vi "meth.PushCluster.vi"(0 "class.GLue in":refnum<class "class.GLue.lvclass">, 7 "Cluster":variant, 11 "error in":errorcluster) -> (4 "class.GLue out":refnum<class "class.GLue.lvclass">, 8 "Pushed?":bool=TRUE, 15 "error out":errorcluster)   [LabVIEW 2014, in "GLue.lvlib" / "class.GLue.lvclass"]
uses:
  class.GLue.lvclass
  class.GLue.lvclass/class.GLue.ctl
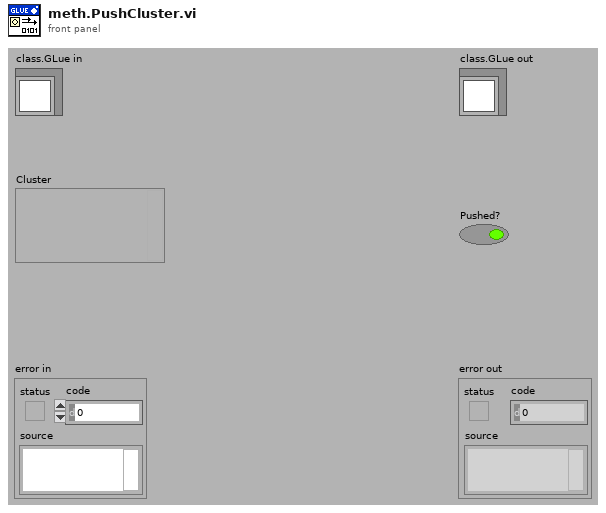
[diagram p1: front panel]
types:
  T1 = cluster{"length":u16, "private":u8, "type":enum8{"<Null>", "I8", "I16", "I32", "I64", "U8", "U16", "U32", "U64", "SGL", "DBL", "EXT", "CSG", "CDB", "CXT", "0x0F", "0x10", "0x11", "0x12", "0x13", "0x14", "Enum U8", "Enum U16", "Enum U32", "Enum U64", "SGL PQ", "DBL PQ", "EXT PQ", "CSG PQ", "CDB PQ", "CXT PQ", "0x1F", "0x20", "Boolean", "0x22", "0x23", "0x24", "0x25", "0x26", "0x27", "0x28", "0x29", "0x2A", "0x2B", "0x2C", "0x2D", "0x2E", "0x2F", "String", "0x31", "Path", "Pict", "0x34", "0x35", "0x36", "DAQ", "0x38", "0x39", "0x3A", "0x3B", "0x3C", "0x3D", "0x3E", "0x3F", "Array", "0x41", "0x42", "0x43", "0x44", "0x45", "0x46", "0x47", "0x48", "0x49", "0x4A", "0x4B", "0x4C", "0x4D", "0x4E", "0x4F", "Cluster", "0x51", "0x52", "Variant", "Waveform", "0x55", "0x56", "0x57", "0x58", "0x59", "0x5A", "0x5B", "0x5C", "0x5D", "0x5E", "0x5F", "0x60", "0x61", "0x62", "0x63", "0x64", "0x65", "0x66", "0x67", "0x68", "0x69", "0x6A", "0x6B", "0x6C", "0x6D", "0x6E", "0x6F", "Refnum"}, "# elements":u16}
  T2 = enum8{"<Null>", "I8", "I16", "I32", "I64", "U8", "U16", "U32", "U64", "SGL", "DBL", "EXT", "CSG", "CDB", "CXT", "0x0F", "0x10", "0x11", "0x12", "0x13", "0x14", "Enum U8", "Enum U16", "Enum U32", "Enum U64", "SGL PQ", "DBL PQ", "EXT PQ", "CSG PQ", "CDB PQ", "CXT PQ", "0x1F", "0x20", "Boolean", "0x22", "0x23", "0x24", "0x25", "0x26", "0x27", "0x28", "0x29", "0x2A", "0x2B", "0x2C", "0x2D", "0x2E", "0x2F", "String", "0x31", "Path", "Pict", "0x34", "0x35", "0x36", "DAQ", "0x38", "0x39", "0x3A", "0x3B", "0x3C", "0x3D", "0x3E", "0x3F", "Array", "0x41", "0x42", "0x43", "0x44", "0x45", "0x46", "0x47", "0x48", "0x49", "0x4A", "0x4B", "0x4C", "0x4D", "0x4E", "0x4F", "Cluster", "0x51", "0x52", "Variant", "Waveform", "0x55", "0x56", "0x57", "0x58", "0x59", "0x5A", "0x5B", "0x5C", "0x5D", "0x5E", "0x5F", "0x60", "0x61", "0x62", "0x63", "0x64", "0x65", "0x66", "0x67", "0x68", "0x69", "0x6A", "0x6B", "0x6C", "0x6D", "0x6E", "0x6F", "Refnum"}
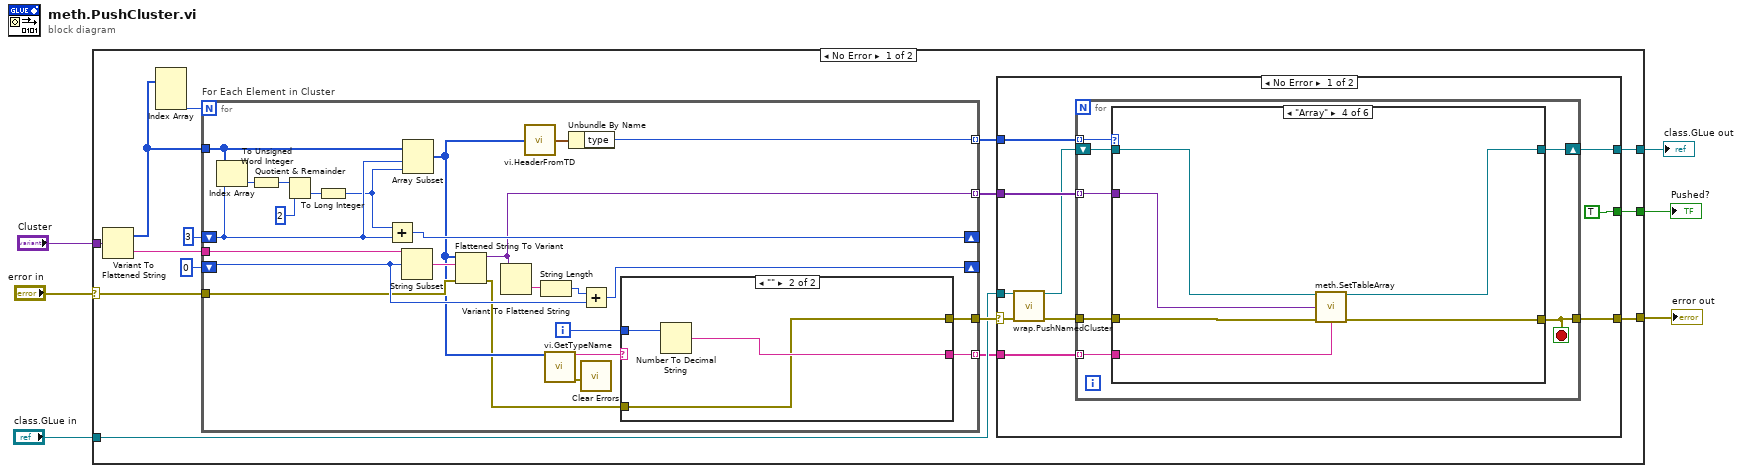
[diagram p0: block diagram]
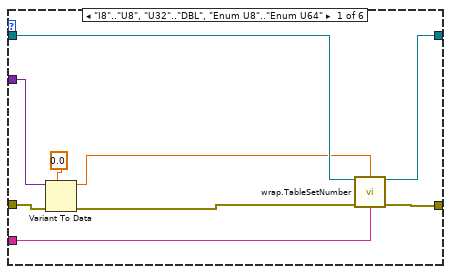
[diagram p2: hidden frame]
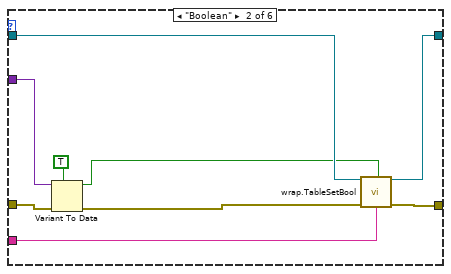
[diagram p3: hidden frame]
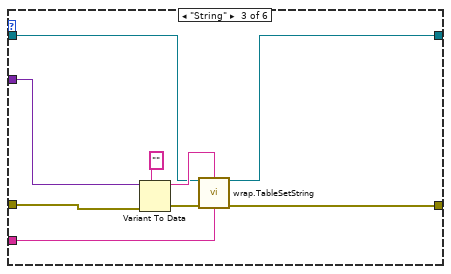
[diagram p4: hidden frame]
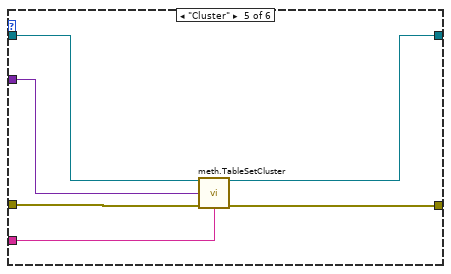
[diagram p5: hidden frame]
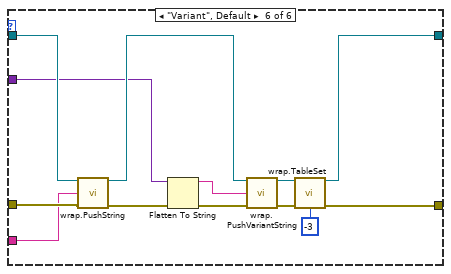
[diagram p6: hidden frame]
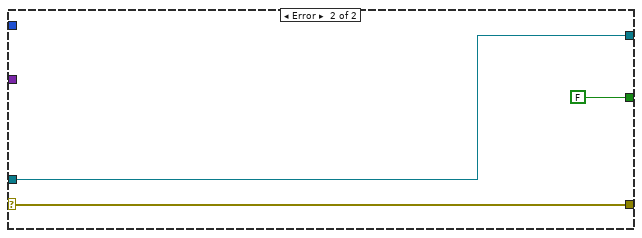
[diagram p7: hidden frame]
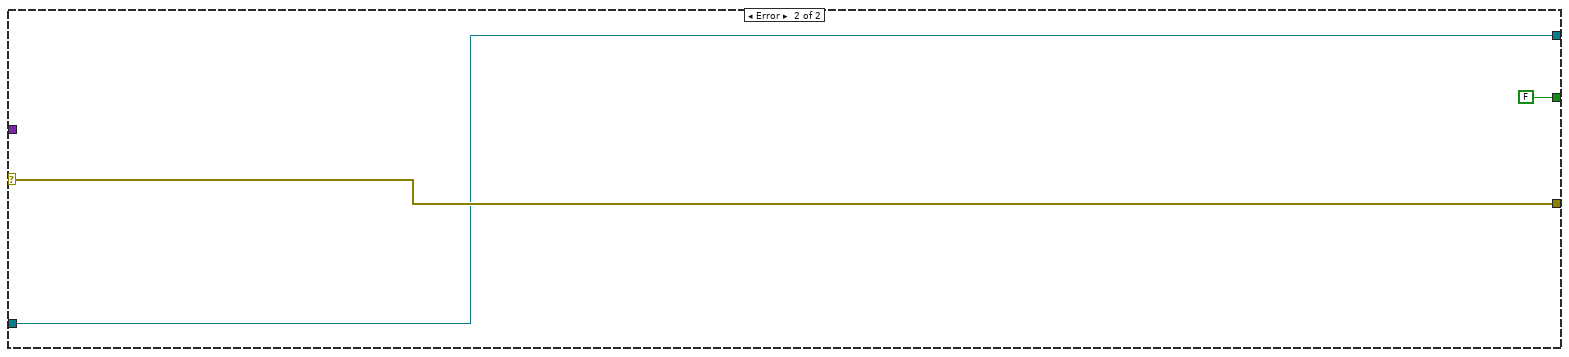
[diagram p9: hidden frame]
diagram:
  n1 = case shown="No Error" "error in" {
    selector: "error in" -> [w15 w126]
    tunnel: [w8 w126] -> w6
    tunnel: [w11 w125] -> w4
    tunnel: "class.GLue in" -> [w12 w125]
    tunnel: "Cluster" -> [w21 _]
    tunnel: [w7 FALSE] -> w1
    frame No Error {
      n2 = Variant To Flattened String(Variant=w21) -> (data string=w16:string, 1:w18:i16[])
      n3 = Index Array(array=w18) -> (element #3=w19:i16)  [unwired: 3 in, 2 out]
      n4 = for "For Each Element in Cluster" {
        N: w19 -> [_]
        shift-right: [w117] -> _
        shift-left: 3 ("Offset past Cluster TD Header") -> [w116]
        tunnel: w18 -> [w118]
        shift-right: [w105] -> _
        shift-left: 0 -> [w106]
        tunnel: w16 -> [w107]
        tunnel: w15 -> [w104]
        tunnel: [w103] -> w14 mode=indexing
        tunnel: [w95] -> w13
        tunnel: [w96] -> w10 mode=indexing
        tunnel: [w100] -> w9 mode=indexing
        i -> [w94]
        n5 = Index Array(array=w118, index=w116) -> (element=w114:i16)
        n6 = To Unsigned Word Integer(number=w114) -> (unsigned 16bit integer=w112:u16)
        n7 = Quotient & Remainder(x=w112, y=u16 2 ("bytes per I16")) -> (floor(x/y)=w115:u16)  [unwired: 1 out]
        n8 = To Long Integer(number=w115) -> (32bit integer=w111:i32)
        n9 = Add(x=w111, y=w116) -> (x+y=w117:i32)
        n10 = String Subset(string=w107, offset (0)=w106) -> (substring=w109:string)  [unwired: 1 in]
        n11 = Array Subset(array=w118, index=w116, length=w111) -> (w102:i16[])
        n12 = Flattened String To Variant(4:w104, 6:w109, 7:w102) -> (0:w97:errorcluster, 3:w103:variant)
        n13 = Variant To Flattened String(Variant=w103) -> (data string=w108:string)  [unwired: 1 out]
        n14 = call "vi.HeaderFromTD.vi"("Type Descriptor"=w102) -> ("Type Descriptor Header"=w101:T1)  [unwired: 4 in]
        n15 = String Length(string=w108) -> (length=w110:i32)
        n16 = call "vi.GetTypeName.vi"("Type Descriptor"=w102) -> ("Name"=w98:string, "error out"=w99:errorcluster)  [unwired: 13 in]
        n17 = Unbundle By Name(w101) -> ("type"=w100:T2)
        n18 = Add(x=w110, y=w106) -> (x+y=w105:i32)
        n19 = call <vilib>:"Clear Errors.vi"("error in (no error)"=w99) -> ()  [unwired: 5 in, 2 out]
        n20 = case shown="\"\"" w98 {
          selector: w98 -> [w120 _]
          tunnel: w97 -> [w119 w121]
          tunnel: [w120 w122] -> w96
          tunnel: [w119 w121] -> w95
          tunnel: w94 -> [_ w123]
          frame Default {
          }
          frame "" {
            n21 = Number To Decimal String(number=w123) -> (decimal integer string=w122:string)  [unwired: 1 in]
          }
        }
      }
      n22 = case shown="No Error" w13 {
        selector: w13 -> [w23 w93]
        tunnel: w14 -> [w31 _]
        tunnel: [w27 w93] -> w8
        tunnel: w12 -> [w25 w92]
        tunnel: [w30 w92] -> w11
        tunnel: w10 -> [w28 _]
        tunnel: w9 -> [w29 _]
        tunnel: [TRUE FALSE] -> w7
        frame No Error {
          n23 = call "wrap.PushNamedCluster.vi"("class.GLue in"=w25, "error in (no error)"=w23) -> ("class.GLue out"=w24:refnum<class "class.GLue.lvclass">, "error out"=w22:errorcluster)  [unwired: 12 in]
          n24 = for {
            tunnel: w31 -> [w33] mode=indexing
            tunnel: w22 -> [w35]
            shift-right: [w36] -> w30
            shift-left: w24 -> [w37]
            tunnel: w29 -> [w38] mode=indexing
            tunnel: w28 -> [w34] mode=indexing
            tunnel: [w32] -> w27
            stop <- w32 stop-if-true
            n25 = case shown="\"Array\"" w38 {
              tunnel: w37 -> [w42 w56 w60 w71 w75 w82]
              tunnel: [w41 w55 w59 w70 w74 w84] -> w36
              tunnel: w35 -> [w47 w53 w62 w69 w77 w80]
              tunnel: [w43 w54 w61 w68 w76 w87] -> w32
              tunnel: w34 -> [w39 w48 w58 w66 w72 w78]
              tunnel: w33 -> [w46 w51 w57 w67 w73 w79]
              frame "I8".."U8", "U32".."DBL", "Enum U8".."Enum U64" {
                n26 = Variant To Data(error in=w47, type=0.0, Variant=w46) -> (data=w40:dbl, error out=w44:errorcluster)
                n27 = call "wrap.TableSetNumber.vi"("class.GLue in"=w42, "Number"=w40, "error in (no error)"=w44, "Name"=w39) -> ("class.GLue out"=w41:refnum<class "class.GLue.lvclass">, "error out"=w43:errorcluster)  [unwired: 10 in]
              }
              frame "Boolean" {
                n28 = Variant To Data(error in=w53, type=TRUE, Variant=w51) -> (data=w49:bool, error out=w52:errorcluster)
                n29 = call "wrap.TableSetBool.vi"("class.GLue in"=w56, "Boolean"=w49, "error in (no error)"=w52, "Name"=w48) -> ("class.GLue out"=w55:refnum<class "class.GLue.lvclass">, "error out"=w54:errorcluster)  [unwired: 10 in]
              }
              frame "String" {
                n30 = Variant To Data(error in=w62, type="", Variant=w57) -> (data=w64:string, error out=w63:errorcluster)
                n31 = call "wrap.TableSetString.vi"("class.GLue in"=w60, "String"=w64, "error in (no error)"=w63, "Name"=w58) -> ("class.GLue out"=w59:refnum<class "class.GLue.lvclass">, "error out"=w61:errorcluster)  [unwired: 10 in]
              }
              frame "Array" {
                n32 = call "meth.SetTableArray.vi"("class.GLue in"=w71, "Array"=w67, "error in (no error)"=w69, "Name"=w66) -> ("class.GLue out"=w70:refnum<class "class.GLue.lvclass">, "error out"=w68:errorcluster)  [unwired: 10 in]
              }
              frame "Cluster" {
                n33 = call "meth.TableSetCluster.vi"("class.GLue in"=w75, "Cluster"=w73, "error in (no error)"=w77, "Name"=w72) -> ("class.GLue out"=w74:refnum<class "class.GLue.lvclass">, "error out"=w76:errorcluster)  [unwired: 10 in]
              }
              frame "Variant", Default {
                n34 = call "wrap.PushString.vi"("class.GLue in"=w82, "String"=w78, "error in (no error)"=w80) -> ("class.GLue out"=w81:refnum<class "class.GLue.lvclass">, "error out"=w83:errorcluster)  [unwired: 11 in]
                n35 = Flatten To String(anything=w79, error in (no error)=w83) -> (data string=w90:string, error out=w89:errorcluster)  [unwired: 2 in, 1 out]
                n36 = call "wrap.PushVariantString.vi"("class.GLue in"=w81, "VariantString"=w90, "error in (no error)"=w89) -> ("class.GLue out"=w85:refnum<class "class.GLue.lvclass">, "error out"=w88:errorcluster)  [unwired: 11 in]
                n37 = call "wrap.TableSet.vi"("class.GLue in"=w85, "error in (no error)"=w88, "Index"=-3) -> ("class.GLue out"=w84:refnum<class "class.GLue.lvclass">, "error out"=w87:errorcluster)  [unwired: 11 in]
              }
            }
          }
        }
        frame Error {
        }
      }
    }
    frame Error {
    }
  }
  "error out" <- w6
  "class.GLue out" <- w4
  "Pushed?" <- w1
